vi "Define other language.vi"(8 "error in (no error)":errorcluster) -> (0 "error out":errorcluster, 2 "cancelled?":bool=TRUE, 3 "language out":string)   [LabVIEW 2012, in "ServiceManager.lvclass"]
uses:
  ServiceManager.lvclass
  <vilib>/Utility/file.llb/Write To Spreadsheet File (string).vi
panel:
  in  "button:cancel":bool
  in  "button:ok":bool
  in  "Command line parameters":string="build\\\\%s.exe \"id=%s\""
  in  "Language":string
  # "This is where to find the executable and how to call it at its ID. \nE.g. for Matlab, it find the executable at the the 'build' directory and can set the ID with extra quotation marks:\n\n build\\\\%s.exe \"id=%s\""
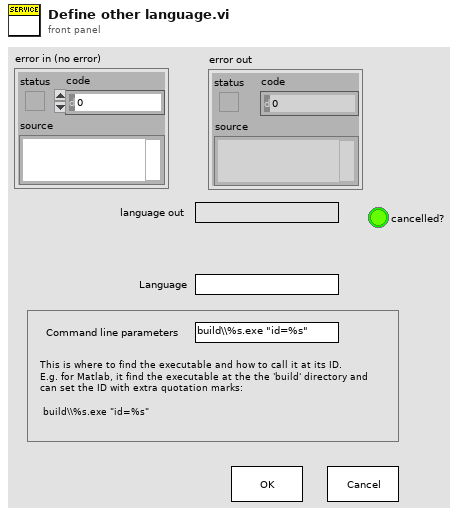
[diagram p1: front panel]
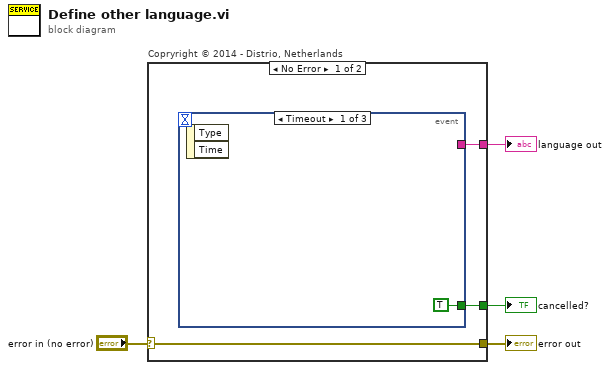
[diagram p0: block diagram]
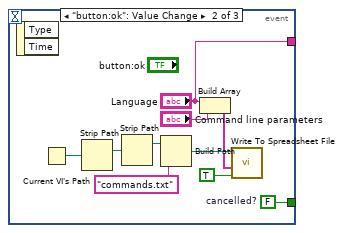
[diagram p2: hidden frame]
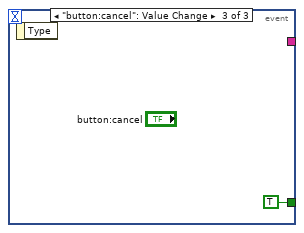
[diagram p3: hidden frame]
diagram:
  n1 = case "Copryright © 2014 - Distrio, Netherlands" shown="No Error" "error in (no error)" {
    selector: "error in (no error)" -> [w5 w20]
    tunnel: [w7 _] -> w4
    tunnel: [w6 _] -> w3
    tunnel: [w5 w20] -> w1
    frame No Error {
      n2 = event shown="[0] Timeout" {
        selector: _ -> [_ _ _]
        dyn-events: _ -> [_ _ _]
        timeout: _ -> [_ _ _]
        tunnel: [_ "Language" _] -> w7
        tunnel: [TRUE ("cancelled?") w9 TRUE ("cancelled?")] -> w6
        event Timeout {
          n3 = event-data() -> ()  [unwired: 1 in, 2 out]
        }
        event "button:ok": Value Change {
          w9 = FALSE  # cancelled?
          n4 = event-data() -> ()  [unwired: 1 in, 2 out]
          n5 = Current VI's Path() -> (path=w15:path)
          n6 = Strip Path(path=w15) -> (stripped path=w16:path)  [unwired: 1 out]
          n7 = Strip Path(path=w16) -> (stripped path=w18:path)  [unwired: 1 out]
          n8 = Build Path(base path=w18, name or relative path="commands.txt") -> (appended path=w13:path)
          n9 = Build Array("Language", "Command line parameters") -> (w12:string[])
          n10 = call-poly <vilib>:"Write To Spreadsheet File.vi"("append to file? (new file:F)"=TRUE, "1D data"=w12, "file path (dialog if empty)"=w13) -> ()  [unwired: 5 in, 1 out]
        }
        event "button:cancel": Value Change {
          n11 = event-data() -> ()  [unwired: 1 in, 1 out]
        }
      }
    }
    frame Error {
    }
  }
  "error out" <- w1
  "language out" <- w4
  "cancelled?" <- w3
